vi "摄像头调试工具.vi"() -> ()   [LabVIEW 2018]
uses:
  <vilib>/userdefined/High Color/IMAQdx.ctl
  <vilib>/vision/Image Controls.llb/IMAQ Image.ctl
  <vilib>/vision/driver/NI_Vision_Acquisition_Software.lvlib
panel:
  in  "视频质量":i32=-1
  out "标题":string="LabVIEW\n视频监控软件"
  out "ID":string
  in  "视频路径":path=path "E:/视频.avi"
  out "image":T1(plugin-control) caption="图像显示区域"
  in  "帧率":u32=10
  in  "录制":bool
  out "时间:":string
  in  "退出":bool
  in  "拍摄":bool
  in  "图片路径":path=path "E:/"
  in  "摄像头:":T2
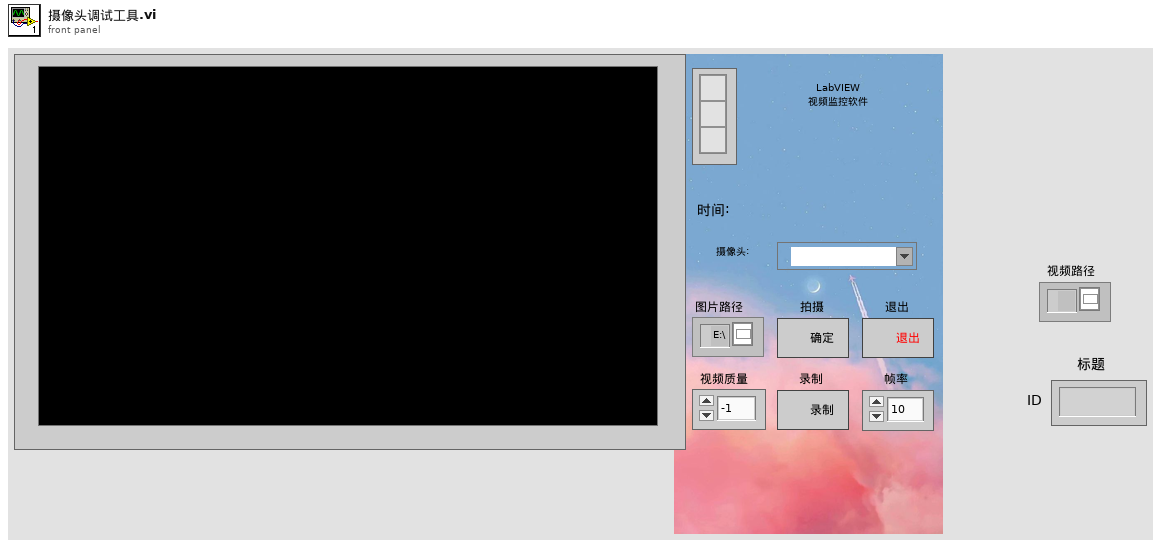
[diagram p1: front panel]
types:
  T1 = typedef "IMAQ Image.ctl" = refnum<image>
  T2 = typedef "IMAQdx.ctl" = refnum<k21>
  T3 = typedef "IMAQ AVI2 Refnum.ctl" = refnum<k20>
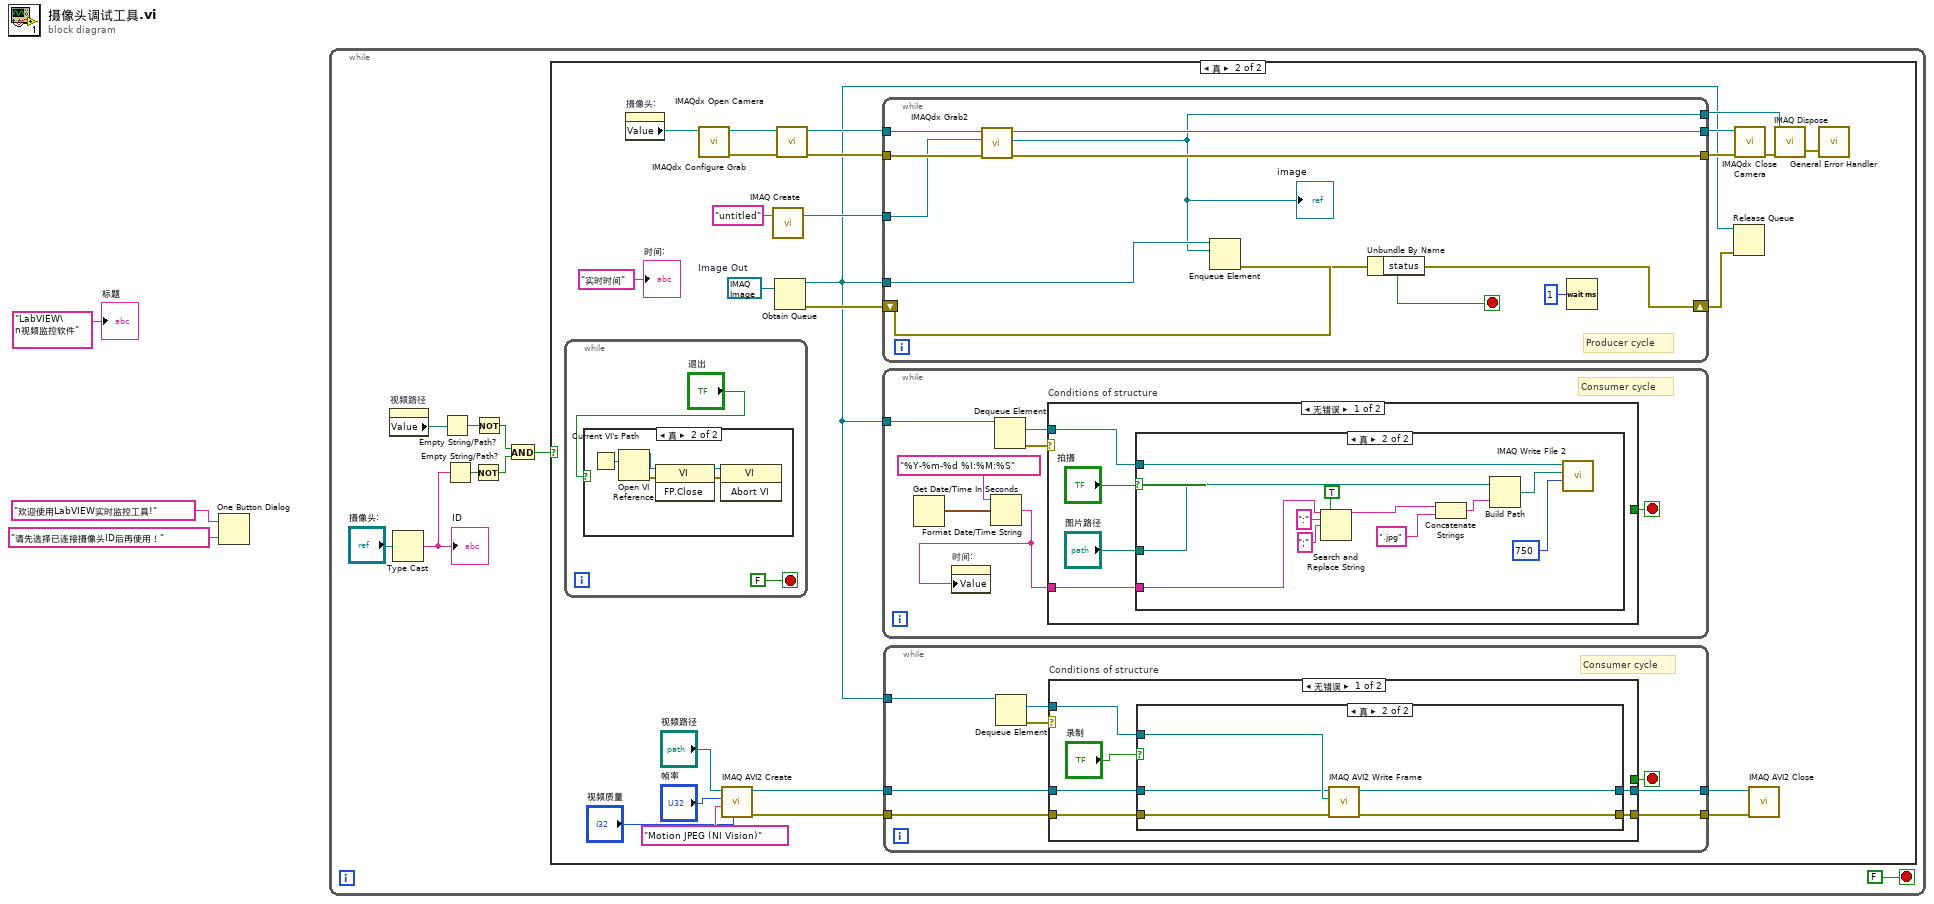
[diagram p0: block diagram]
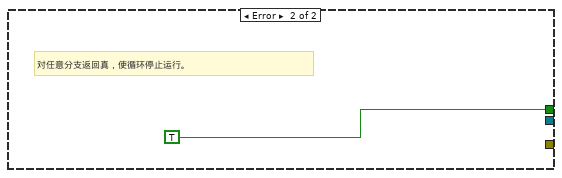
[diagram p5: hidden frame]
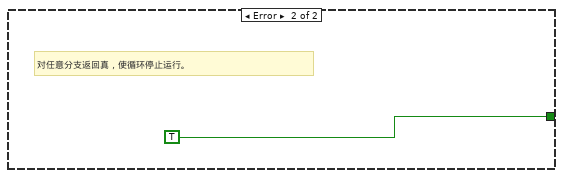
[diagram p7: hidden frame]
diagram:
  n1 = One Button Dialog(message="欢迎使用LabVIEW实时监控工具!" ("消息"), button name ("OK")="请先选择已连接摄像头ID后再使用！" ("按钮名称（“确定”）")) -> ()  [unwired: 1 out]
  n2 = while {
    stop <- FALSE stop-if-true
    n3 = property on="视频路径" class="Path"() -> ("Value"=w8:path)  [unwired: 2 in, 2 out]
    n4 = Type Cast(x="摄像头:") -> (*(type *) &x=w11:string)  [unwired: 1 in]
    "ID" <- w11
    n5 = Empty String/Path?(string/path=w8) -> (empty?=w7:bool)
    n6 = Empty String/Path?(string/path=w11) -> (empty?=w10:bool)
    n7 = Not(x=w10) -> (.not. x?=w5:bool)
    n8 = Not(x=w7) -> (.not. x?=w6:bool)
    n9 = And(x=w6, y=w5) -> (x .and. y?=w4:bool)
    n10 = case shown="真" w4 {
      frame False {
      }
      frame True {
        w25 = T1 refnum  # Image Out
        n11 = while {
          stop <- FALSE stop-if-true
          n12 = case shown="真" "退出" {
            frame False {
            }
            frame True {
              n13 = Current VI's Path() -> (path=w44:path)
              n14 = Open VI Reference(vi path=w44) -> (vi reference=w43:refnum<vi>, error out=w42:errorcluster)  [unwired: 5 in]
              n15 = invoke class="VI" method="FP.Close"(reference=w43, error in=w42) -> (reference out=w40:refnum<vi>, error out=w41:errorcluster)  [unwired: 1 in, 1 out]
              n16 = invoke class="VI" method="Abort VI"(reference=w40, error in=w41) -> ()  [unwired: 1 in, 3 out]
            }
          }
        }
        n17 = property on="摄像头:" class="IMAQdx (严格)"() -> ("Value"=w22:T2)  [unwired: 2 in, 2 out]
        n18 = call <vilib>:"IMAQdx Open Camera.vi"("Session In"=w22) -> ("error out"=w37:errorcluster, "Session Out"=w36:T2)  [unwired: 9 in]
        n19 = call "IMAQ AVI2 Create"("Quality"="视频质量", "Codec"="Motion JPEG (NI Vision)", "Frames Per Second"="帧率", "AVI Path"="视频路径") -> ("error out"=w17:errorcluster, "AVI Refnum"=w18:T3)  [unwired: 6 in]
        n20 = call "IMAQ Create"("Image Name"="untitled") -> ("New Image"=w24:T1)  [unwired: 4 in, 1 out]
        n21 = Obtain Queue(element data type=w25) -> (queue out=w23:refnum<queue>, error out=w34:errorcluster)  [unwired: 4 in, 1 out]
        n22 = call <vilib>:"IMAQdx Configure Grab.vi"("error in"=w37, "Session In"=w36) -> ("error out"=w31:errorcluster, "Session Out"=w32:T2)  [unwired: 8 in]
        n23 = while {
          shift-right: [w96] -> w33
          shift-left: w34 -> [w97]
          tunnel: w23 -> [w98]
          tunnel: w32 -> [w95]
          tunnel: w31 -> [w94]
          tunnel: [w93] -> w30
          tunnel: [w88] -> w29
          tunnel: [w92] -> w26
          tunnel: w24 -> [w91]
          stop <- w90 stop-if-true
          # "Producer cycle"
          n24 = call <vilib>:"IMAQdx Grab2.vi"("error in"=w94, "Image In"=w91, "Session In"=w95) -> ("error out"=w92:errorcluster, "Image Out"=w88:T1, "Session Out"=w93:T2)  [unwired: 5 in, 1 out]
          "image" <- w88
          n25 = Enqueue Element(queue=w98, element=w88, error in (no error)=w97) -> (error out=w96:errorcluster)  [unwired: 1 in, 2 out]
          n26 = Unbundle By Name(w96) -> ("status"=w90:bool)
          n27 = Wait (ms)(milliseconds to wait=u32 1 ("等待时间（毫秒）")) -> ()  [unwired: 1 out]
        }
        n28 = while {
          tunnel: w23 -> [w71]
          stop <- w69 stop-if-true
          # "Consumer cycle"
          n29 = Get Date/Time In Seconds() -> (seconds since 1Jan1904=w67:timestamp)
          n30 = Format Date/Time String(time format string (%c)="%Y-%m-%d %I:%M:%S" ("时间格式字符串(%c)"), seconds (now)=w67) -> (date/time string=w65:string)  [unwired: 1 in]
          n31 = property on="时间:" class="Str"("Value"=w65) -> ()  [unwired: 2 in, 2 out]
          n32 = Dequeue Element(queue=w71) -> (element=w68:T1, error out=w70:errorcluster)  [unwired: 2 in, 2 out]
          n33 = case "Conditions of structure" shown="无错误" w70 {
            tunnel: w68 -> [w74 _]
            tunnel: [_ TRUE] -> w69
            tunnel: w65 -> [w72 _]
            frame No Error {
              n34 = case shown="真" "拍摄" {
                tunnel: w74 -> [_ w85]
                tunnel: "图片路径" -> [_ w84]
                tunnel: w72 -> [_ w76]
                frame False {
                }
                frame True {
                  n35 = Search and Replace String(replace all?=TRUE ("替换全部？(F)"), input string=w76, search string=":" ("搜索字符串"), replace string=";" ("替换字符串(\"\")")) -> (result string=w77:string)  [unwired: 4 in, 3 out]
                  n36 = Concatenate Strings(w77, ".jpg" ("字符串")) -> (w83:string)
                  n37 = Build Path(base path=w84, name or relative path=w83) -> (appended path=w81:path)
                  n38 = call-poly "IMAQ Write File 2"("Image Quality"=u32 750, "File Path"=w81, "Image"=w85) -> ()  [unwired: 7 in, 2 out]
                }
              }
            }
            frame Error {
              # "对任意分支返回真，使循环停止运行。"
            }
          }
        }
        n39 = while {
          tunnel: w23 -> [w52]
          tunnel: [w48] -> w21
          tunnel: [w47] -> w20
          tunnel: w18 -> [w46]
          tunnel: w17 -> [w45]
          stop <- w50 stop-if-true
          # "Consumer cycle"
          n40 = Dequeue Element(queue=w52) -> (element=w49:T1, error out=w51:errorcluster)  [unwired: 2 in, 2 out]
          n41 = case "Conditions of structure" shown="无错误" w51 {
            tunnel: w49 -> [w58 _]
            tunnel: [_ TRUE] -> w50
            tunnel: [w57 _] -> w48
            tunnel: [w56 _] -> w47
            tunnel: w46 -> [w55 _]
            tunnel: w45 -> [w54 _]
            frame No Error {
              n42 = case shown="真" "录制" {
                tunnel: w58 -> [_ w61]
                tunnel: [_ w63] -> w57
                tunnel: [_ w62] -> w56
                tunnel: w55 -> [_ w60]
                tunnel: w54 -> [_ w59]
                frame False {
                }
                frame True {
                  n43 = call "IMAQ AVI2 Write Frame"("error in (no error)"=w59, "Image"=w61, "AVI Refnum"=w60) -> ("error out"=w62:errorcluster, "AVI Refnum (duplicate)"=w63:T3)  [unwired: 6 in, 1 out]
                }
              }
            }
            frame Error {
              # "对任意分支返回真，使循环停止运行。"
            }
          }
        }
        n44 = Release Queue(queue=w23, error in (no error)=w33) -> ()  [unwired: 1 in, 3 out]
        n45 = call <vilib>:"IMAQdx Close Camera.vi"("error in"=w26, "Session In"=w30) -> ("error out"=w27:errorcluster)  [unwired: 9 in]
        n46 = call "IMAQ AVI2 Close"("error in (no error)"=w20, "AVI Refnum"=w21) -> ()  [unwired: 9 in, 1 out]
        n47 = call "IMAQ Dispose"("Image"=w29, "error in (no error)"=w27) -> ("error out"=w28:errorcluster)  [unwired: 4 in]
        n48 = call <vilib>:"General Error Handler.vi"("error in (no error)"=w28) -> ()  [unwired: 10 in, 5 out]
        "时间:" <- "实时时间" ("时间:")
      }
    }
  }
  "标题" <- "LabVIEW\n视频监控软件" ("标题")
